vi "Timer On Delay（SM).vi"(8 "error in":errorcluster, 10 "preset time (ms)":u32=1000, 11 "input":bool) -> (0 "error out":errorcluster, 2 "elapsed time (ms)":u32, 3 "output":bool)   [LabVIEW 2013, in "毫秒定时器.lvlib"]
uses:
  <vilib>/ptbypt/NI_PtbyPt.lvlib
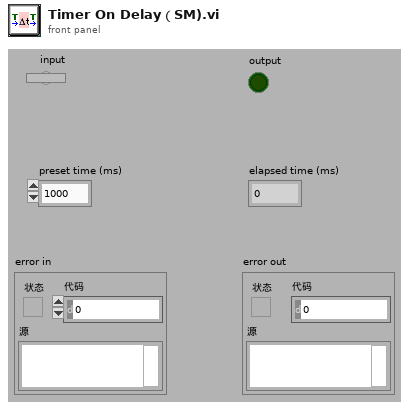
[diagram p1: front panel]
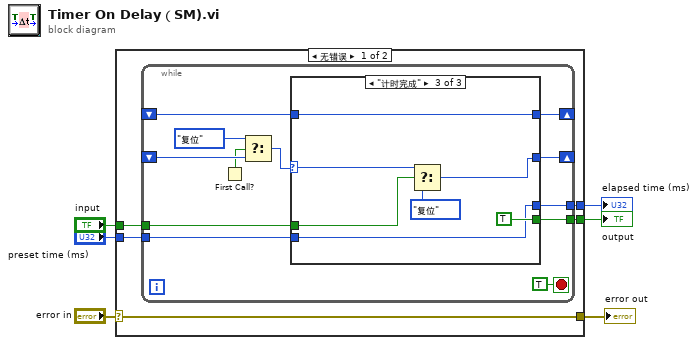
[diagram p0: block diagram]
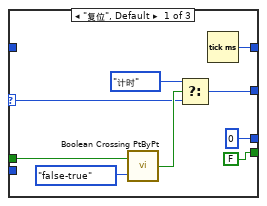
[diagram p2: hidden frame]
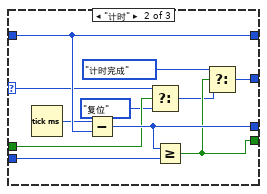
[diagram p3: hidden frame]
diagram:
  n1 = case shown="无错误" "error in" {
    selector: "error in" -> [w11 w51]
    tunnel: [w11 w51] -> w5
    tunnel: [w10 _] -> w4
    tunnel: [w9 _] -> w3
    tunnel: "input" -> [w8 _]
    tunnel: "preset time (ms)" -> [w7 _]
    frame No Error {
      n2 = while {
        shift-right: [w18] -> _
        shift-left: _ -> [w22]
        shift-right: [w17] -> _
        shift-left: _ -> [w16]
        tunnel: [w15] -> w10
        tunnel: [w13] -> w9
        tunnel: w8 -> [w14]
        tunnel: w7 -> [w12]
        stop <- TRUE stop-if-true
        n3 = First Call?() -> (First Call?: T/F=w21:bool)
        n4 = Select(t=enum16{"复位", "计时", "计时完成"}."复位", s=w21, f=w22) -> (s? t:f=w19:enum16{"复位", "计时", "计时完成"})
        n5 = case shown="\"计时完成\"" w19 {
          selector: w19 -> [w26 w38 w46]
          tunnel: [w25 w33 w45] -> w18
          tunnel: [w32 w43 w48] -> w17
          tunnel: w16 -> [_ w43 w48]
          tunnel: [FALSE ("output") w36 TRUE ("output")] -> w15
          tunnel: w14 -> [w30 w39 w47]
          tunnel: [u32 0 ("elapsed time (ms)") w40 w49] -> w13
          tunnel: w12 -> [_ w41 w49]
          frame "复位", Default {
            n6 = call <vilib>:"Boolean Crossing PtByPt.vi"("direction"=enum16{"either", "false-true", "true-false"}."false-true", "input"=w30) -> ("crossing"=w28:bool)  [unwired: 1 in]
            n7 = Select(t=enum16{"复位", "计时", "计时完成"}."计时", s=w28, f=w26) -> (s? t:f=w25:enum16{"复位", "计时", "计时完成"})
            n8 = Tick Count (ms)() -> (millisecond timer value=w32:u32)
          }
          frame "计时" {
            n9 = Tick Count (ms)() -> (millisecond timer value=w42:u32)
            n10 = Subtract(x=w42, y=w43) -> (x-y=w40:u32)
            n11 = Select(t=w38, s=w39, f=enum16{"复位", "计时", "计时完成"}."复位") -> (s? t:f=w34:enum16{"复位", "计时", "计时完成"})
            n12 = Greater Or Equal?(x=w40, y=w41) -> (x >= y?=w36:bool)
            n13 = Select(t=enum16{"复位", "计时", "计时完成"}."计时完成" ("f"), s=w36, f=w34) -> (s? t:f=w33:enum16{"复位", "计时", "计时完成"})
          }
          frame "计时完成" {
            n14 = Select(t=w46, s=w47, f=enum16{"复位", "计时", "计时完成"}."复位") -> (s? t:f=w45:enum16{"复位", "计时", "计时完成"})
          }
        }
      }
    }
    frame Error {
    }
  }
  "error out" <- w5
  "output" <- w4
  "elapsed time (ms)" <- w3
